vi "NumberFileName.vi"(1 "String":string=".eye", 2 "Digits":i32=3, 3 "File number":i32, 4 "file name":string) -> (0 "Numbered File":string)   [LabVIEW 2022 SP3]
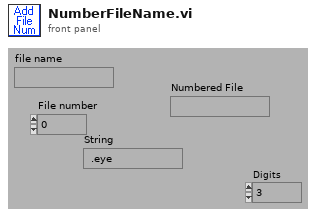
[diagram p1: front panel]
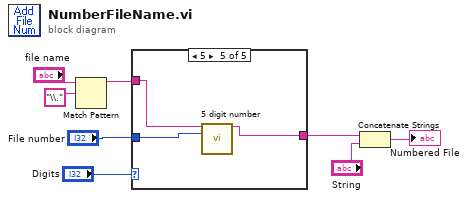
[diagram p0: block diagram]
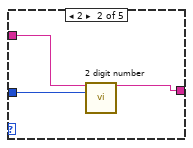
[diagram p3: hidden frame]
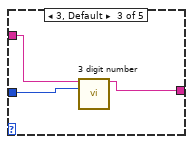
[diagram p4: hidden frame]
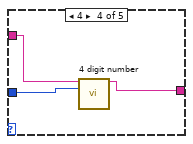
[diagram p5: hidden frame]
diagram:
  n1 = Match Pattern(string="file name", regular expression="\\.") -> (before substring=w5:string)  [unwired: 4 out]
  n2 = case shown="5" "Digits" {
    tunnel: w5 -> [w9 w10 w13 w16 w19]
    tunnel: "File number" -> [_ w11 w15 w18 w21]
    tunnel: [w9 w12 w14 w17 w20] -> w2
    frame 0 {
    }
    frame 2 {
      n3 = call "2 digit number"("Beginning Text"=w10, "num"=w11) -> ("Result"=w12:string)  [unwired: 1 in, 12 out]
    }
    frame 3, Default {
      n4 = call "3 digit number"("Beginning Text"=w13, "num"=w15) -> ("Result"=w14:string)  [unwired: 1 in, 12 out]
    }
    frame 4 {
      n5 = call "4 digit number"("Beginning Text"=w16, "num"=w18) -> ("Result"=w17:string)  [unwired: 1 in, 12 out]
    }
    frame 5 {
      n6 = call "5 digit number"("Beginning Text"=w19, "num"=w21) -> ("Result"=w20:string)  [unwired: 1 in, 12 out]
    }
  }
  n7 = Concatenate Strings(w2, "String") -> (→"Numbered File":string)
